vi "Tools_String Buffer Strings.vi"(6 "Insert between Strings (\"\")":string, 9 "Number of Strings to Buffer":u8=15, 11 "New String":string) -> (3 "Buffered String Series":string)   [LabVIEW 2017]
doc: "This VI buffers and returns a series of strings using a an internal shift register. It is commonly used to display the last N strings returned form a device, instrument, process, etc. The user can select how many strings are buffered and returned from this VI. \n\nThe Insert between Strings parameter value is inserted between each of the buffered strings."
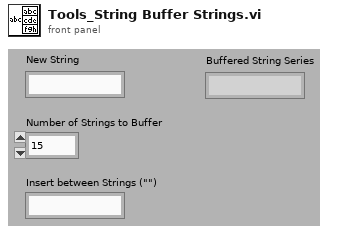
[diagram p1: front panel]
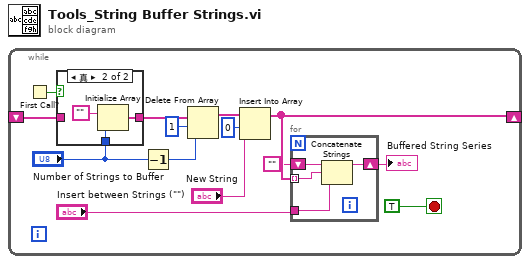
[diagram p0: block diagram]
diagram:
  n1 = while {
    shift-right: [w6] -> _
    shift-left: _ -> [w13]
    stop <- TRUE stop-if-true
    n2 = First Call?() -> (First Call?: T/F=w14:bool)
    n3 = case shown="真" w14 {
      tunnel: [w19 w21] -> w12
      tunnel: w13 -> [w19 _]
      tunnel: "Number of Strings to Buffer" -> [_ w20]
      frame False {
      }
      frame True {
        n4 = Initialize Array("" ("element"), w20) -> (w21:string[])
      }
    }
    n5 = Decrement(x="Number of Strings to Buffer") -> (x-1=w10:u8)
    n6 = Delete From Array(array=w12, length=1, index=w10) -> (array with subset deleted=w8:string[])  [unwired: 1 out]
    n7 = Insert Into Array(array=w8, index=0, new element="New String") -> (w6:string[])
    n8 = for {
      tunnel: w6 -> [w17] mode=indexing
      shift-right: [w16] -> w4
      shift-left: "" ("element") -> [w18]
      tunnel: "Insert between Strings (\"\")" -> [w15]
      n9 = Concatenate Strings(w18, w17, w15) -> (w16:string)
    }
    "Buffered String Series" <- w4
  }
